vi "Wristband main - Pinch Button based.vi"() -> ()   [LabVIEW 2014]
uses:
  Typedef/sensor_data.ctl
  Typedef/flexext_data.ctl
  Typedef/pinch_data.ctl
  SubVIs/Save Blocks - 2D.vi
  <vilib>/MakerHub/LINX/Public/Peripherals/Analog/Analog Read N Chans.vi
  <vilib>/MakerHub/LINX/LMH-LINX.lvlib
panel:
  in  "Pinch medio":bool
  in  "Pinch mignolo":bool
  in  "Pinch anulare":bool
  in  "Pinch indice":bool
  out "Spread":u8
  in  "Spread":bool
  out "Pinch cluster":T1
  in  "Clear Plot":bool
  in  "Acquire":bool
  in  "Tacq":u32=50 min=50 max=10000 step=50 format="%.0fms"
  in  "N pts":i32=500
  in  "Session name":string="Session 0"
  in  "Save to path":path=path "C:/Users/Andrea/Desktop/Progetto Canada/Dati"
  out "Leap \nConnected?":bool=TRUE caption="Leap Motion"
  in  "Arduino Port":refnum<visa-resource-name>="COM20"
  out "Status":bool=TRUE caption="Arduino"
  out "Sensor Chart":T2(graph)={"Sensor  Chan 0"=1.3720703125, "Sensor Chan 2"=1.357421875, "Sensor Chan 4"=1.3525390625, "Sensor Chan 5"=1.3232421875}
  out "Grab Strength":u8
  out "Flexext cluster":T3
  out "Sensor Data":T4={"Sensor  Chan 0"=1.396484375, "Sensor Chan 1"=1.3818359375, "Sensor Chan 2"=1.376953125, "Sensor Chan 3"=1.3818359375, "Sensor Chan 4"=1.38671875, "Sensor Chan 5"=1.357421875}
  in  "Exit":bool
  out "Event Chart":T5(graph)
  # "Connection panel"
  # "Acquisition panel"
  # "Save settings"
  # "Connection status"
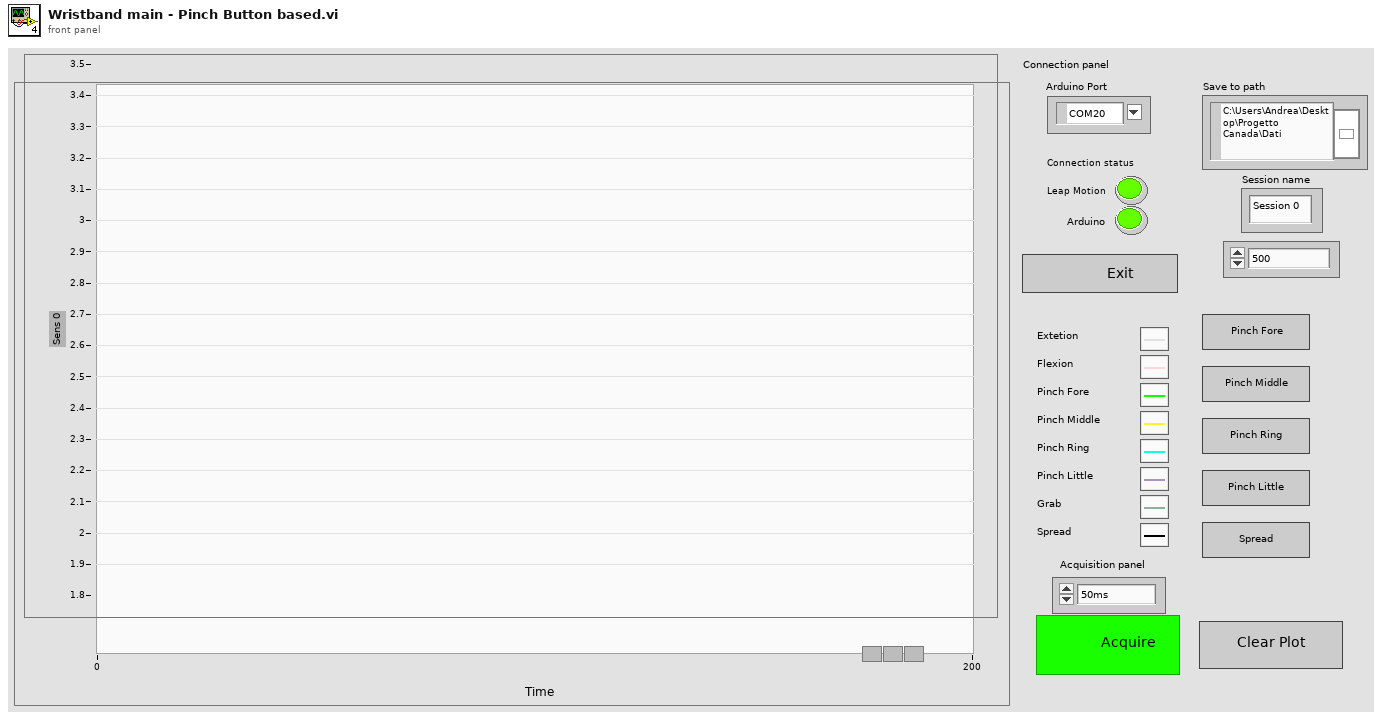
[diagram p1: front panel]
types:
  T1 = typedef "pinch_data.ctl" = cluster{"Indice":u8, "Medio":u8, "Anulare":u8, "Mignolo":u8}
  T2 = cluster{"Sensor  Chan 0":dbl, "Sensor Chan 2":dbl, "Sensor Chan 4":dbl, "Sensor Chan 5":dbl}
  T3 = typedef "flexext_data.ctl" = cluster{"Estensione":u8, "Flessione":u8}
  T4 = typedef "Sensor_data.ctl" = cluster{"Sensor  Chan 0":dbl, "Sensor Chan 1":dbl, "Sensor Chan 2":dbl, "Sensor Chan 3":dbl, "Sensor Chan 4":dbl, "Sensor Chan 5":dbl}
  T5 = cluster{"Estensione":u8, "Flessione":u8, "Pollice":u8, "Indice":u8, "Medio":u8, "Anulare":u8, "Mignolo":u8, "Grab Strength":u8}
  T6 = typedef "LMH-LINX.lvlib/LINX Ref.ctl" = cluster{"Platform":T7, "Interface":T8, "LINX Device Config":T9}
  T7 = typedef "LMH-LINX.lvlib/Platform.ctl" = enum16{"LINX", "myRIO"}
  T8 = typedef "LMH-LINX.lvlib/Interface.ctl" = enum16{"Serial", "TCP"}
  T9 = typedef "LMH-LINX.lvlib/Device.lvlib/LINX Device Config.ctl" = cluster{"Interface":T8, "COM Port":refnum<visa-resource-name>, "TCP Configuration":T10, "Device Family":u8, "Device ID":u8, "Device Name":string, "TCP Ref":refnum<k5>, "Channels":T11}
  T10 = typedef "LMH-LINX.lvlib/Device.lvlib/TCP Config.ctl" = cluster{"IP Address":string, "Port":u16}
  T11 = typedef "LMH-LINX.lvlib/Channels.ctl" = cluster{"DI":u8[], "DO":u8[], "AI":u8[], "AO":u8[], "PWM":u8[], "QE":u8[], "UART":u8[], "I2C 2":u8[], "SPI":u8[], "CAN":u8[], "Servo":u8[], "AI Ref (V)":dbl, "AO Ref (V)":dbl, "AO Resolution (Bits)":u8}
  T12 = typedef "Leap Handle.ctl" = cluster{"LeapCSharp":refnum<k24>}
  T13 = cluster{"Pinch indice ":bool, "Pinch medio ":bool, "Pinch anulare ":bool, "Pinch mignolo ":bool}
  T14 = cluster{"Sensor  Chan 0":dbl, "Sensor Chan 2":dbl, "Sensor Chan 4":dbl, "Sensor Chan 5":dbl}[]
  T15 = cluster{"Estensione":u8, "Flessione":u8, "Pollice":u8, "Indice":u8, "Medio":u8, "Anulare":u8, "Mignolo":u8, "Grab Strength":u8}[]
  T16 = cluster{"Estensione":u8, "Flessione":u8, "Indice":u8, "Medio":u8, "Anulare":u8, "Mignolo":u8, "Grab Strength":u8, "Spread":u8}
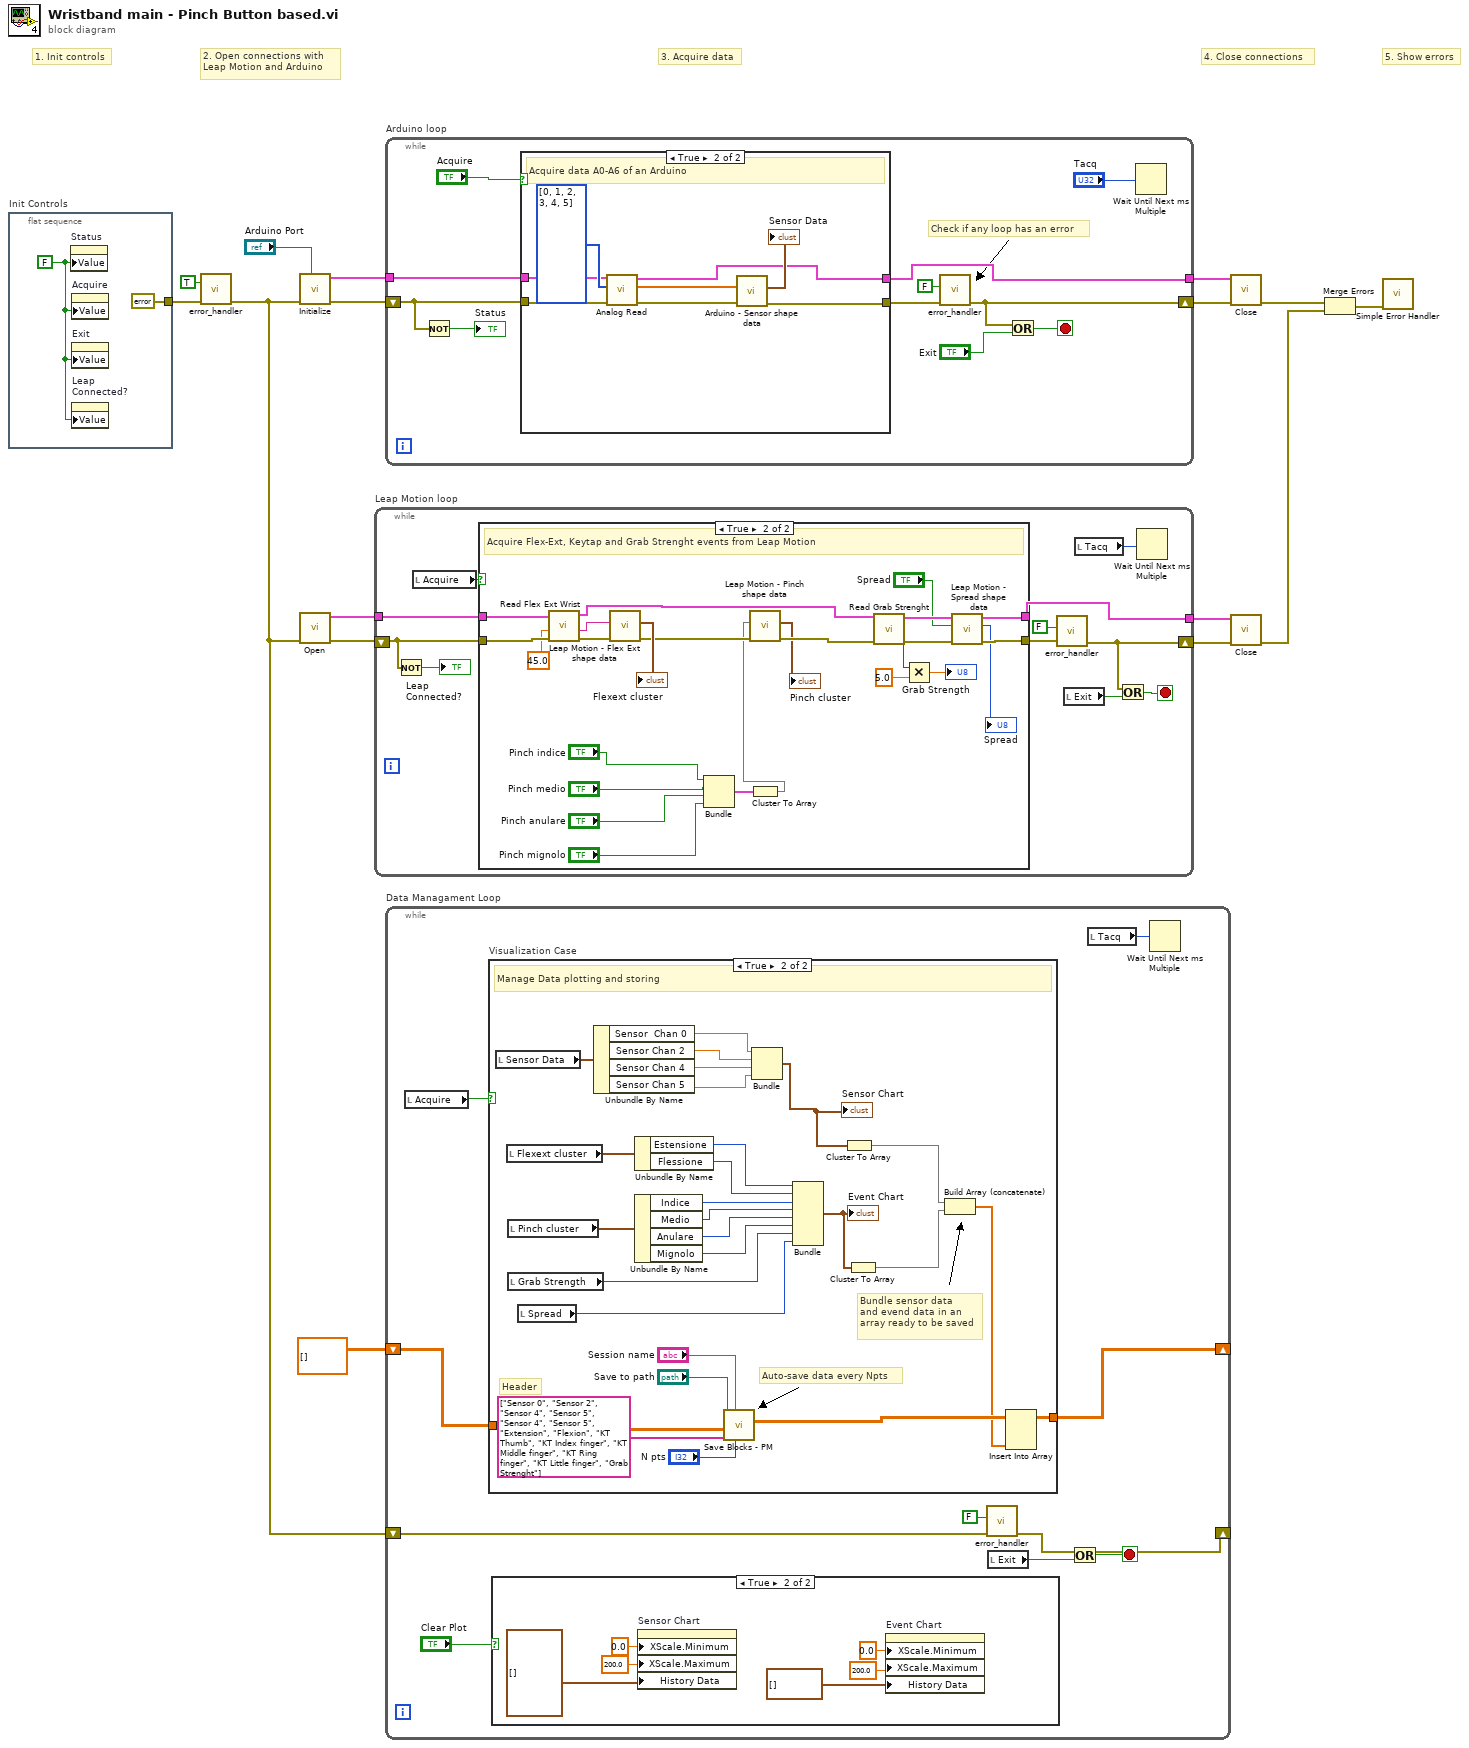
[diagram p0: block diagram]
diagram:
  # "5. Show errors"
  # "4. Close connections"
  # "3. Acquire data"
  # "2. Open connections with\nLeap Motion and Arduino"
  # "1. Init controls"
  n1 = flat-sequence "Init Controls" {
    tunnel: [errorcluster {"status"=FALSE, "code"=0, "source"=""} ("Error In")] -> w7
    frame #0 {
      w17 = FALSE ("Status")
      n2 = property on="Status" class="Bool (strict)"("Value"=w17) -> ()  [unwired: 2 in, 2 out]
      n3 = property on="Acquire" class="Bool (strict)"("Value"=w17) -> ()  [unwired: 2 in, 2 out]
      n4 = property on="Exit" class="Bool (strict)"("Value"=w17) -> ()  [unwired: 2 in, 2 out]
      n5 = property on="Leap \nConnected?" class="Bool (strict)"("Value"=w17) -> ()  [unwired: 2 in, 2 out]
    }
  }
  n6 = call "error_handler.vi"("Error In"=w7, "Reset"=TRUE) -> ("Error Out"=w6:errorcluster)  [unwired: 9 in]
  n7 = call <vilib>:"Initialize.vi"("Serial Port"="Arduino Port", "Error In"=w6) -> ("Error Out"=w15:errorcluster, "LINX Ref"=w16:T6)  [unwired: 7 in, 1 out]
  n8 = call "Open.vi"("Error In"=w6) -> ("Error Out"=w10:errorcluster, "Leap Handle"=w11:T12)  [unwired: 9 in]
  n9 = while "Leap Motion loop" {
    tunnel: w11 -> [w27]
    tunnel: [w21] -> w9
    shift-right: [w23] -> w8
    shift-left: w10 -> [w20]
    stop <- w28 stop-if-true
    n10 = Not(x=w20) -> (.not. x?=→"Leap \nConnected?":bool)
    n11 = local read "Acquire"() -> (w25:bool)
    n12 = case shown="True" w25 {
      tunnel: w27 -> [w31 w55]
      tunnel: w20 -> [w30 w54]
      tunnel: [w31 w49] -> w21
      tunnel: [w30 w42] -> w24
      frame False {
        # "Idle"
      }
      frame True {
        # "Acquire Flex-Ext, Keytap and Grab Strenght events from Leap Motion"
        n13 = call "Read Flex Ext Wrist.vi"("Error In"=w54, "Flex Extension threshold"=sgl 45.0, "Leap Handle In"=w55) -> ("Error Out"=w52:errorcluster, "Wrist Flextion/Extension"=w51:string, "Leap Handle Out"=w39:T12)  [unwired: 4 in]
        n14 = call "Leap Motion - Flex Ext shape data.vi"("Error In"=w52, "Event In"=w51) -> ("Error Out"=w38:errorcluster, "Flexext cluster"=→"Flexext cluster":T3)  [unwired: 8 in]
        n15 = Bundle("Pinch indice"="Pinch indice", "Pinch medio"="Pinch medio", "Pinch anulare"="Pinch anulare", "Pinch mignolo"="Pinch mignolo") -> (w33:T13)  [unwired: 1 in]
        n16 = Cluster To Array(cluster=w33) -> (array=w32:bool[])
        n17 = call "Leap Motion - Pinch shape data.vi"("Error In"=w38, "Pinch"=w32) -> ("Error Out"=w45:errorcluster, "Pinch cluster"=→"Pinch cluster":T1)  [unwired: 8 in]
        n18 = call "Read Grab Strenght.vi"("Error In"=w45, "Leap Handle In"=w39) -> ("Error Out"=w43:errorcluster, "Numeric Palm State"=w46:i32, "Leap Handle Out"=w49:T12)  [unwired: 5 in, 2 out]
        n19 = Multiply(x=w46, y=sgl 5.0) -> (x*y=→"Grab Strength":sgl)
        n20 = call "Leap Motion - Spread shape data.vi"("Error In"=w43, "Spread  Button 2"="Spread") -> ("Error Out"=w42:errorcluster, "Spread"=→"Spread":u8)  [unwired: 8 in]
      }
    }
    n21 = call "error_handler.vi"("Error In"=w24, "Reset"=FALSE) -> ("Error Out"=w23:errorcluster)  [unwired: 9 in]
    n22 = local read "Exit"() -> (w29:bool)
    n23 = local read "Tacq"() -> (w26:u32)
    n24 = Or(x=w23, y=w29) -> (x .or. y?=w28:bool)
    n25 = Wait Until Next ms Multiple(millisecond multiple=w26) -> ()  [unwired: 1 out]
  }
  n26 = while "Arduino loop" {
    tunnel: w16 -> [w65]
    tunnel: [w57] -> w12
    shift-right: [w58] -> w13
    shift-left: w15 -> [w61]
    stop <- w63 stop-if-true
    # "Check if any loop has an error"
    n27 = Not(x=w61) -> (.not. x?=→"Status":bool)
    n28 = case shown="True" "Acquire" {
      tunnel: w65 -> [w67 w74]
      tunnel: w61 -> [w68 w76]
      tunnel: [w67 w69] -> w57
      tunnel: [w68 w72] -> w59
      frame False {
        # "Idle"
      }
      frame True {
        # "Acquire data A0-A6 of an Arduino"
        n29 = call-poly <vilib>:"Analog Read.vi"("Error In"=w76, "AI Channel(s)"=u8[] [0, 1, 2, 3, 4, 5], "LINX Resource"=w74) -> ("Error Out"=w73:errorcluster, "Voltages"=w71:dbl[], "LINX Resource"=w69:T6)  [unwired: 5 in, 1 out]
        n30 = call "Arduino - Sensor shape data.vi"("Error In"=w73, "Sensor Data in"=w71) -> ("Error Out"=w72:errorcluster, "Sensor Data Out"=→"Sensor Data":T4)  [unwired: 8 in]
      }
    }
    n31 = call "error_handler.vi"("Error In"=w59, "Reset"=FALSE) -> ("Error Out"=w58:errorcluster)  [unwired: 9 in]
    n32 = Or(x=w58, y="Exit") -> (x .or. y?=w63:bool)
    n33 = Wait Until Next ms Multiple(millisecond multiple="Tacq") -> ()  [unwired: 1 out]
  }
  n34 = while "Data Managament Loop" {
    shift-right: [w81] -> _
    shift-left: w6 -> [w82]
    shift-right: [w80] -> _
    shift-left: dbl[][] [] -> [w79]
    stop <- w83 stop-if-true
    n35 = local read "Acquire"() -> (w86:bool)
    n36 = case "Visualization Case" shown="True" w86 {
      tunnel: [w93 w112] -> w80
      tunnel: w79 -> [w93 w110]
      frame False {
        # "Idle"
      }
      frame True {
        # "Header"
        # "Auto-save data every Npts"
        # "Bundle sensor data\nand evend data in an\narray ready to be saved"
        # "Manage Data plotting and storing"
        n37 = local read "Sensor Data"() -> (w108:T4)
        n38 = local read "Flexext cluster"() -> (w120:T3)
        n39 = local read "Pinch cluster"() -> (w102:T1)
        n40 = local read "Grab Strength"() -> (w97:u8)
        n41 = local read "Spread"() -> (w96:u8)
        n42 = Unbundle By Name(w108) -> ("Sensor  Chan 0"=w107:dbl, "Sensor Chan 2"=w106:dbl, "Sensor Chan 4"=w105:dbl, "Sensor Chan 5"=w104:dbl)
        n43 = Unbundle By Name(w120) -> ("Estensione"=w119:u8, "Flessione"=w118:u8)
        n44 = Unbundle By Name(w102) -> ("Indice"=w101:u8, "Medio"=w100:u8, "Anulare"=w99:u8, "Mignolo"=w98:u8)
        n45 = call-poly "Save Blocks - PM.vi"("N pts"="N pts", "Session name"="Session name", "2D Data In"=w110, "Column headers"=string[] ["Sensor 0", "Sensor 2", "Sensor 4", "Sensor 5", "Sensor 4", "Sensor 5", "Extension", "Flexion", "KT Thumb", "KT Index finger", "KT Middle finger", "KT Ring finger", "KT Little finger", "Grab Strenght"], "Save to path"="Save to path") -> ("2D Data Out"=w116:dbl[][])  [unwired: 5 in, 1 out]
        n46 = Bundle("Sensor  Chan 0"=w107, "Sensor Chan 2"=w106, "Sensor Chan 4"=w105, "Sensor Chan 5"=w104) -> (w103:T2)  [unwired: 1 in]
        "Sensor Chart" <- w103
        n47 = Bundle("Estensione"=w119, "Flessione"=w118, "Indice"=w101, "Medio"=w100, "Anulare"=w99, "Mignolo"=w98, "Grab Strength"=w97, "Spread"=w96) -> (w95:T16)  [unwired: 1 in]
        "Event Chart" <- w95
        n48 = Cluster To Array(cluster=w103) -> (array=w117:dbl[])
        n49 = Cluster To Array(cluster=w95) -> (array=w94:u8[])
        n50 = Build Array (concatenate)(w117, w94) -> (w111:dbl[])
        n51 = Insert Into Array(array=w116, new element=w111) -> (w112:dbl[][])  [unwired: 2 in]
      }
    }
    n52 = case shown="True" "Clear Plot" {
      frame False {
      }
      frame True {
        n53 = property on="Sensor Chart" class="WFChart (strict)"("XScale.Minimum"=0.0 ("X Scale.Range:Minimum"), "XScale.Maximum"=200.0 ("X Scale.Range:Maximum"), "History Data"=T14 []) -> ()  [unwired: 2 in, 2 out]
        n54 = property on="Event Chart" class="WFChart (strict)"("XScale.Minimum"=0.0 ("X Scale.Range:Minimum"), "XScale.Maximum"=200.0 ("X Scale.Range:Maximum"), "History Data"=T15 []) -> ()  [unwired: 2 in, 2 out]
      }
    }
    n55 = call "error_handler.vi"("Error In"=w82, "Reset"=FALSE) -> ("Error Out"=w81:errorcluster)  [unwired: 9 in]
    n56 = local read "Exit"() -> (w84:bool)
    n57 = Or(x=w81, y=w84) -> (x .or. y?=w83:bool)
    n58 = local read "Tacq"() -> (w78:u32)
    n59 = Wait Until Next ms Multiple(millisecond multiple=w78) -> ()  [unwired: 1 out]
  }
  n60 = call <vilib>:"Close.vi"("Error In"=w13, "LINX Resource"=w12) -> ("Error Out"=w3:errorcluster)  [unwired: 8 in, 1 out]
  n61 = call <vilib>:"Close.vi"("Error In"=w8, "Leap Handle"=w9) -> ("Error Out"=w2:errorcluster)  [unwired: 9 in]
  n62 = Merge Errors(w3, w2) -> (w4:errorcluster)
  n63 = call <vilib>:"Simple Error Handler.vi"("error in (no error)"=w4) -> ()  [unwired: 4 in, 5 out]
